vi "Load Variant from JSON File.vi"(8 "error in":errorcluster, 11 "file path":path) -> (0 "error out":errorcluster, 3 "Variant out":variant)   [LabVIEW 2017, in "Variant JSON API.lvlib"]
doc: "Loads a JSON instance from the given file."
uses:
  Variant JSON API.lvlib
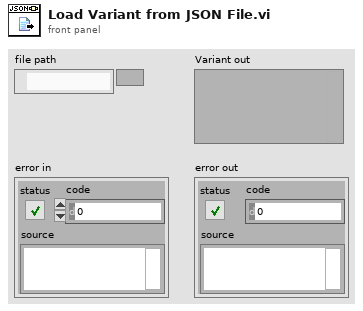
[diagram p1: front panel]
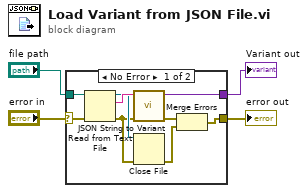
[diagram p0: block diagram]
diagram:
  n1 = case shown="No Error" "error in" {
    selector: "error in" -> [w5 w14]
    tunnel: [w13 _] -> w4
    tunnel: "file path" -> [w10 _]
    tunnel: [w6 w14] -> w2
    frame No Error {
      n2 = Read from Text File(file (use dialog)=w10, error in=w5) -> (refnum out=w11:refnum<file>, text=w12:string, error out=w9:errorcluster)  [unwired: 2 in, 1 out]
      n3 = call "JSON String to Variant.vi"("error in (no error)"=w9, "JSON String"=w12) -> ("error out"=w8:errorcluster, "Variant out"=w13:variant)  [unwired: 8 in]
      n4 = Close File(refnum=w11, error in=w9) -> (error out=w7:errorcluster)  [unwired: 1 out]
      n5 = Merge Errors(w8, w7) -> (w6:errorcluster)
    }
    frame Error {
    }
  }
  "Variant out" <- w4
  "error out" <- w2
